vi "Soll-Ist_Prüfung.vi"(9 "Index":i32, 10 "Istwerte Ref.":refnum<vi>[](array[refnum])) -> (0 "Fehler":bool, 1 "Istwert":sgl[](array[numeric]))   [LabVIEW 2020, in "Erweiterte Konfig.lvlib" / "CG-Check Konfig.lvlib"]
uses:
  CG-Check Konfig.lvlib
  Aktion_CG-Check.ctl
  Messdaten/Aktionen FGV Messdaten.ctl
  Messdaten/Gewichtung (Stichprobe).ctl
  Messdaten/Messdaten.lvlib
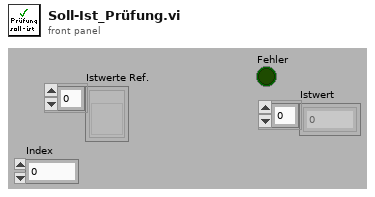
[diagram p1: front panel]
types:
  T1 = typedef "Messdaten.lvlib/Aktionen FGV Messdaten.ctl" = enum16{"lesen", "schreiben", "löschen", "Mittelwerte", "Komponente"}
  T2 = typedef "Erweiterte Konfig.lvlib/CG-Check Konfig.lvlib/Aktion_CG-Check.ctl" = enum16{"lesen", "schreiben", "laden", "Komponente", "Aktive?", "speichern"}
  T3 = cluster{"Aufschaltdauer":sgl, "Prüfdauer":sgl, "Mittelwertanzahl":u8}
  T4 = typedef "Messdaten.lvlib/Gewichtung (Stichprobe).ctl" = enum16{"Sample", "Population"}
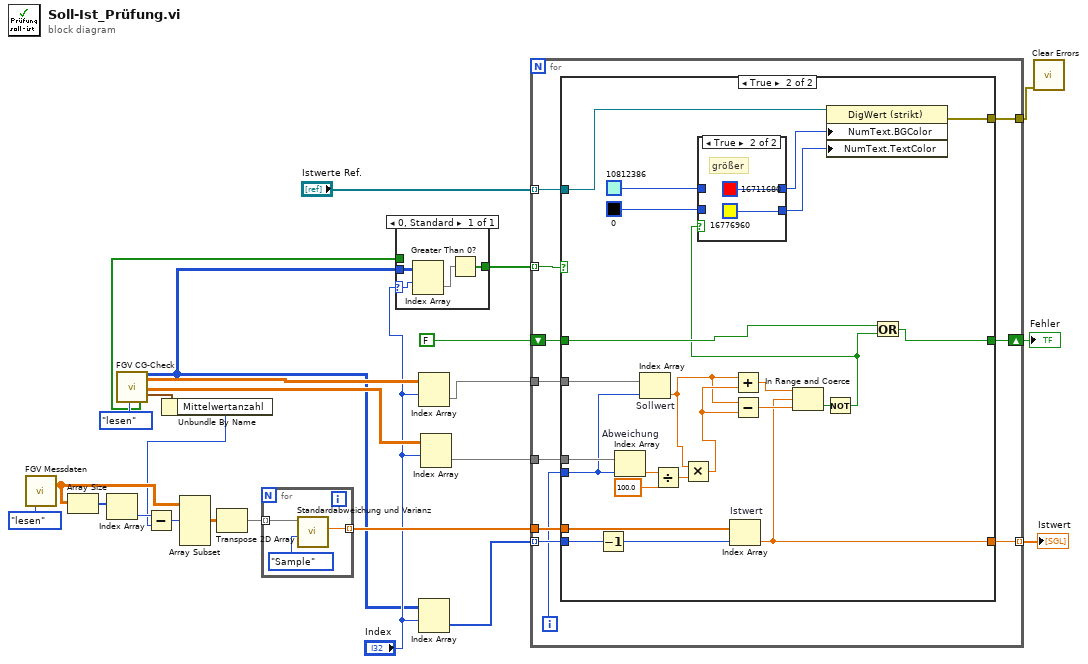
[diagram p0: block diagram]
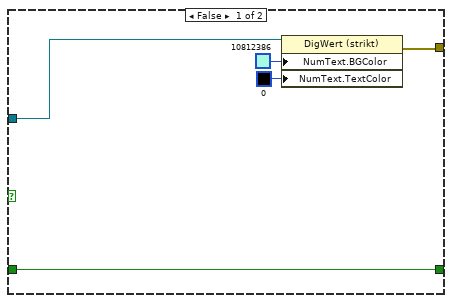
[diagram p2: hidden frame]
diagram:
  n1 = call "FGV Messdaten.vi"("Aktionen"=Aktionen_FGV_Messdaten."lesen") -> ("Messdaten"=w17:sgl[][])  [unwired: 6 in, 8 out]
  n2 = Array Size(array=w17) -> (size(s)=w19:i32[])
  n3 = Index Array(array=w19) -> (element=w20:i32)  [unwired: 1 in]
  n4 = call "FGV CG-Check.vi"("Aktion"=Aktion_CG-Check."lesen") -> ("Aktive?"=w4:bool[], "Komponenten"=w1:u16[][], "Sollwerte"=w7:sgl[][], "max Abweichung"=w9:sgl[][], "Cluster"=w11:T3)  [unwired: 11 in, 3 out]
  n5 = Unbundle By Name(w11) -> ("Mittelwertanzahl"=w10:u8)
  n6 = Subtract(x=w20, y=w10) -> (x-y=w21:i32)
  n7 = Array Subset(array=w17, index (row)=w21) -> (w22:sgl[][])  [unwired: 3 in]
  n8 = Transpose 2D Array(2D array=w22) -> (transposed array=w18:sgl[][])
  n9 = for {
    tunnel: [w27] -> w16 mode=indexing
    tunnel: w18 -> [w26] mode=indexing
    n10 = call "Standardabweichung und Varianz.vi"("Gewichtung (Stichprobe)"=Gewichtung_(Stichprobe)."Sample", "X"=w26) -> ("Mittelwert"=w27:sgl)  [unwired: 7 in, 2 out]
  }
  n11 = case shown="0, Standard" "Index" {
    selector: "Index" -> [w32]
    tunnel: w4 -> [_]
    tunnel: [w29] -> w2
    tunnel: w1 -> [w31]
    frame 0, Default {
      n12 = Index Array(array=w31, index (row)=w32) -> (element=w30:u16[])  [unwired: 1 in]
      n13 = Greater Than 0?(x=w30) -> (x > 0?=w29:bool[])
    }
  }
  n14 = Index Array(array=w7, index (row)="Index") -> (element=w6:sgl[])  [unwired: 1 in]
  n15 = Index Array ("Istwert")(array=w1, index (row)="Index") -> (element=w5:u16[])  [unwired: 1 in]
  n16 = Index Array(array=w9, index (row)="Index") -> (element=w8:sgl[])  [unwired: 1 in]
  n17 = for {
    tunnel: w16 -> [w43]
    tunnel: w6 -> [w37]
    tunnel: w8 -> [w42]
    tunnel: [w41] -> w24 mode=indexing
    shift-right: [w35] -> w14
    shift-left: FALSE -> [w40]
    tunnel: "Istwerte Ref." -> [w39] mode=indexing
    tunnel: [w38] -> w12
    tunnel: w5 -> [w36] mode=indexing
    tunnel: w2 -> [w33] mode=indexing
    i -> [w34]
    n18 = case shown="True" w33 {
      tunnel: w43 -> [_ w72]
      tunnel: w42 -> [_ w71]
      tunnel: [_ w67] -> w41
      tunnel: w40 -> [w48 w66]
      tunnel: w39 -> [w47 w62]
      tunnel: [w46 w61] -> w38
      tunnel: w37 -> [_ w55]
      tunnel: w36 -> [_ w52]
      tunnel: [w48 w50] -> w35
      tunnel: w34 -> [_ w49]
      frame False {
        n19 = property class="DigWert (strikt)"(reference=w47, "NumText.BGColor"=u32 10812386 ("Hintergrund"), "NumText.TextColor"=u32 0 ("Hintergrund")) -> (error out=w46:errorcluster)  [unwired: 1 in, 1 out]
      }
      frame True {
        n20 = Decrement(x=w52) -> (x-1=w60:u16)
        n21 = Index Array "Abweichung"(array=w71, index=w49) -> (element=w59:sgl)
        n22 = Index Array "Sollwert"(array=w55, index=w49) -> (element=w54:sgl)
        n23 = Divide(x=w59, y=sgl 100.0) -> (x/y=w57:sgl)
        n24 = Multiply(x=w54, y=w57) -> (x*y=w56:sgl)
        n25 = Index Array "Istwert"(array=w72, index=w60) -> (element=w67:sgl)
        n26 = Add(x=w54, y=w56) -> (x+y=w69:sgl)
        n27 = Subtract(x=w54, y=w56) -> (x-y=w70:sgl)
        n28 = In Range and Coerce(upper limit=w69, x=w67, lower limit=w70) -> (In Range?=w68:bool)  [unwired: 1 out]
        n29 = Not(x=w68) -> (.not. x?=w51:bool)
        n30 = case shown="True" w51 {
          tunnel: u32 10812386 ("Hintergrund") -> [w74 _]
          tunnel: [w74 u32 16711680 ("Hintergrund")] -> w64
          tunnel: u32 0 ("Hintergrund") -> [w73 _]
          tunnel: [w73 u32 16776960 ("Hintergrund")] -> w65
          frame False {
          }
          frame True {
            # "größer"
          }
        }
        n31 = property class="DigWert (strikt)"(reference=w62, "NumText.BGColor"=w64, "NumText.TextColor"=w65) -> (error out=w61:errorcluster)  [unwired: 1 in, 1 out]
        n32 = Or(x=w66, y=w51) -> (x .or. y?=w50:bool)
      }
    }
  }
  "Fehler" <- w14
  "Istwert" <- w24
  n33 = call <vilib>:"Clear Errors.vi"("error in (no error)"=w12) -> ()  [unwired: 5 in, 2 out]
